vi "Read Config File.vi"(8 "error in (no error)":errorcluster, 11 "System Actor in":refnum<class "System Actor.lvclass">) -> (0 "error out":errorcluster, 2 "Ref":T1, 3 "System Actor out":refnum<class "System Actor.lvclass">)   [LabVIEW 2024, in "System Actor.lvclass"]
uses:
  System Actor.lvclass
  <vilib>/Utility/config.llb/Config Data RefNum.ctl
  System Actor.lvclass/System Actor.ctl
  <vilib>/Utility/config.llb/NI_LVConfig.lvlib
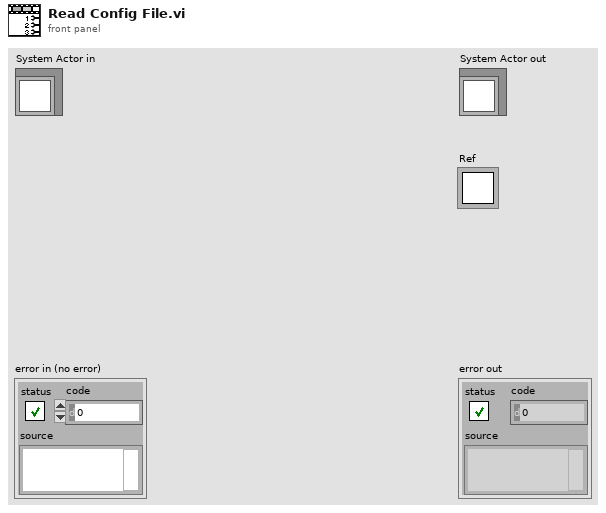
[diagram p1: front panel]
types:
  T1 = typedef "NI_LVConfig.lvlib/Config Data RefNum.ctl" = refnum<k1>
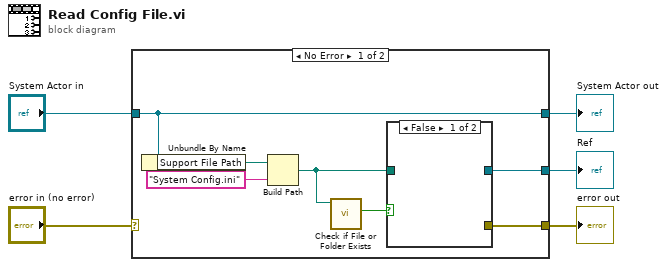
[diagram p0: block diagram]
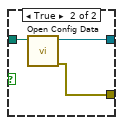
[diagram p2: hidden frame]
diagram:
  n1 = case shown="No Error" "error in (no error)" {
    selector: "error in (no error)" -> [_ w17]
    tunnel: [w9 w17] -> w4
    tunnel: [w12 w16] -> w2
    tunnel: "System Actor in" -> [w12 w16]
    tunnel: [w8 _] -> w1
    frame No Error {
      n2 = Unbundle By Name(w12) -> ("Support File Path"=w11:path)
      n3 = Build Path(base path=w11, name or relative path="System Config.ini") -> (appended path=w7:path)
      n4 = call <vilib>:"Check if File or Folder Exists.vi"("path"=w7) -> ("file or folder exists?"=w6:bool)  [unwired: 8 in, 2 out]
      n5 = case shown="False" w6 {
        tunnel: [_ w15] -> w9
        tunnel: [_ w14] -> w8
        tunnel: w7 -> [_ w13]
        frame False {
        }
        frame True {
          n6 = call <vilib>:"Open Config Data.vi"("configuration file path"=w13) -> ("error out"=w15:errorcluster, "refnum"=w14:T1)  [unwired: 8 in, 1 out]
        }
      }
    }
    frame Error {
    }
  }
  "error out" <- w4
  "System Actor out" <- w2
  "Ref" <- w1
